vi "TCP Data Client.vi"() -> ()   [LabVIEW 2015]
uses:
  <vilib>/measure/maspectr.llb/FFT Power Spectrum and PSD for 1 Chan (CDB).vi
  <vilib>/measure/NI_MAPro.lvlib
panel:
  in  "fs":dbl format="%#_6p"
  out "Power Spectrum / PSD":cluster{"f0":dbl, "df":dbl, "magnitude":dbl[]}(graph)
  in  "Server Closed":string="The server VI closed the connection."
  in  "Stop":bool
  out "Receveived IQ signal":dbl[][](graph)
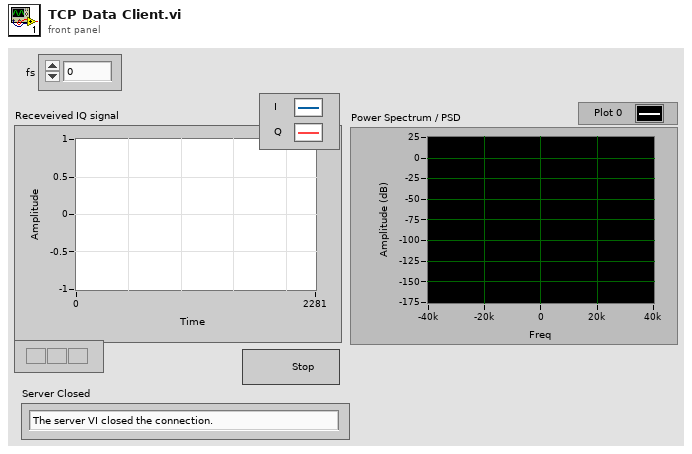
[diagram p1: front panel]
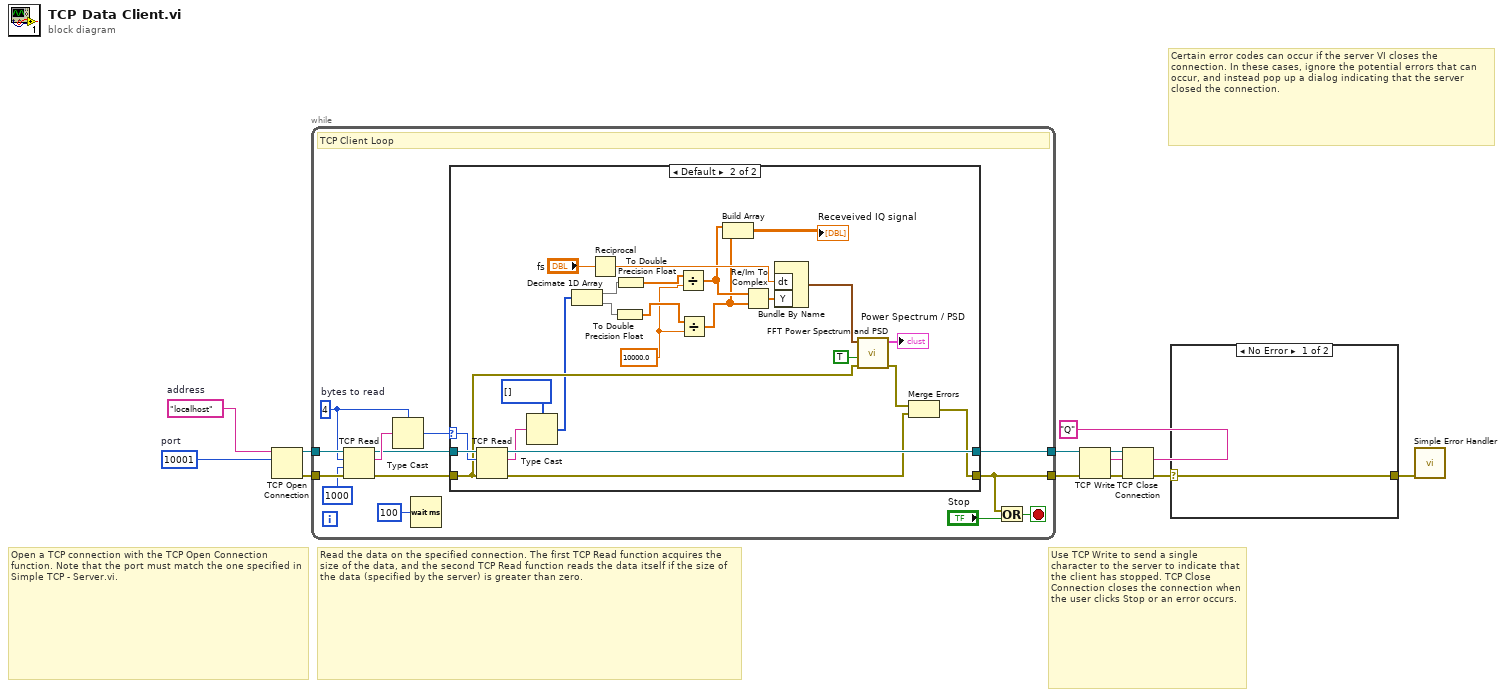
[diagram p0: block diagram]
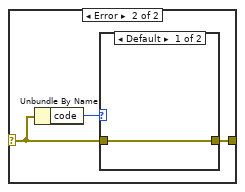
[diagram p2: hidden frame]
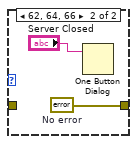
[diagram p3: hidden frame]
diagram:
  w1 = u16 10001  # port
  w2 = "localhost"  # address
  # "Certain error codes can occur if the server VI closes the connection. In these cases, ignore the potential errors that can occur, and instead pop up a dialog indicating that the server closed the connection."
  # "Use TCP Write to send a single character to the server to indicate that the client has stopped. TCP Close Connection closes the connection when the user clicks Stop or an error occurs."
  # "Read the data on the specified connection. The first TCP Read function acquires the size of the data, and the second TCP Read function reads the data itself if the size of the data (specified by the server) is greater than zero."
  # "Open a TCP connection with the TCP Open Connection function. Note that the port must match the one specified in Simple TCP - Server.vi."
  n1 = TCP Open Connection(address=w2, remote port or service name=w1) -> (connection ID=w11:refnum<k5>, error out=w10:errorcluster)  [unwired: 3 in]
  n2 = while {
    tunnel: w10 -> [w20]
    tunnel: w11 -> [w21]
    tunnel: [w15] -> w8
    tunnel: [w14] -> w6
    stop <- w17 stop-if-true
    w19 = 4  # bytes to read
    # "TCP Client Loop"
    n3 = TCP Read(connection ID=w21, bytes to read=w19, error in (no error)=w20, 9:1000 ("timeout ms (25000)")) -> (connection ID out=w23:refnum<k5>, data out=w24:string, error out=w22:errorcluster)  [unwired: 1 in]
    n4 = Type Cast(type=w19, x=w24) -> (*(type *) &x=w13:i32)
    n5 = Wait (ms)(milliseconds to wait=u32 100) -> ()  [unwired: 1 out]
    n6 = case shown="Default" w13 {
      selector: w13 -> [_ w46]
      tunnel: w23 -> [w26 w50]
      tunnel: w22 -> [w25 w43]
      tunnel: [w26 w48] -> w15
      tunnel: [w25 w40] -> w14
      frame ..0 {
        # "The server has not written any data"
      }
      frame Default {
        w29 = 10000.0
        n7 = TCP Read(connection ID=w50, bytes to read=w46, error in (no error)=w43) -> (connection ID out=w48:refnum<k5>, data out=w47:string, error out=w41:errorcluster)  [unwired: 2 in]
        n8 = Type Cast(type=i16[] [] ("chart"), x=w47) -> (*(type *) &x=w39:i16[])
        n9 = Decimate 1D Array(w39) -> (w34:i16[], w33:i16[])
        n10 = Reciprocal(x="fs") -> (1/x=w37:dbl)
        n11 = To Double Precision Float(number=w33) -> (double precision float=w30:dbl[])
        n12 = To Double Precision Float(number=w34) -> (double precision float=w31:dbl[])
        n13 = Divide(x=w31, y=w29) -> (x/y=w28:dbl[])
        n14 = Divide(x=w30, y=w29) -> (x/y=w27:dbl[])
        n15 = Build Array(w28, w27) -> (→"Receveived IQ signal":dbl[][])
        n16 = Re/Im To Complex(1:w27, 2:w28) -> (0:w38:cdb[])
        n17 = Bundle By Name("dt"=w37, "Y"=w38) -> (w35:waveform(cdb))  [unwired: 1 in]
        n18 = call-poly <vilib>:"FFT Power Spectrum and PSD.vi"("error in (no error)"=w43, "dB On (F)"=TRUE, "time signal"=w35) -> ("error out"=w42:errorcluster, "Power Spectrum / PSD"=→"Power Spectrum / PSD":cluster{"f0":dbl, "df":dbl, "magnitude":dbl[]})  [unwired: 5 in, 2 out]
        n19 = Merge Errors(w42, w41) -> (w40:errorcluster)
      }
    }
    n20 = Or(x=w14, y="Stop") -> (x .or. y?=w17:bool)
  }
  n21 = TCP Write(connection ID=w8, data in="Q", error in (no error)=w6) -> (connection ID out=w9:refnum<k5>, error out=w7:errorcluster)  [unwired: 2 out]
  n22 = TCP Close Connection(connection ID=w9, error in (no error)=w7) -> (error out=w4:errorcluster)  [unwired: 1 in, 1 out]
  n23 = case shown="No Error" w4 {
    selector: w4 -> [w51 w53]
    tunnel: [w51 w52] -> w3
    frame No Error {
    }
    frame Error {
      n24 = Unbundle By Name(w53) -> ("code"=w54:i32)
      n25 = case shown="Default" w54 {
        tunnel: w53 -> [w55 _]
        tunnel: [w55 w57] -> w52
        frame Default {
        }
        frame 62, 64, 66 {
          w57 = errorcluster {"status"=FALSE, "code"=0, "source"=""}  # No error
          n26 = One Button Dialog(message="Server Closed") -> ()  [unwired: 1 in, 1 out]
        }
      }
    }
  }
  n27 = call <vilib>:"Simple Error Handler.vi"("error in (no error)"=w3) -> ()  [unwired: 4 in, 5 out]
